vi "move.vi"(8 "error in":errorcluster, 9 "Relative? (T)":bool=TRUE, 10 "Destination (steps)":i16, 11 "Picomotor in":refnum<class "Picomotor.lvclass">) -> (0 "error out":errorcluster, 3 "Picomotor out":refnum<class "Picomotor.lvclass">)   [LabVIEW 2020, in "Picomotor.lvclass"]
uses:
  Picomotor.lvclass
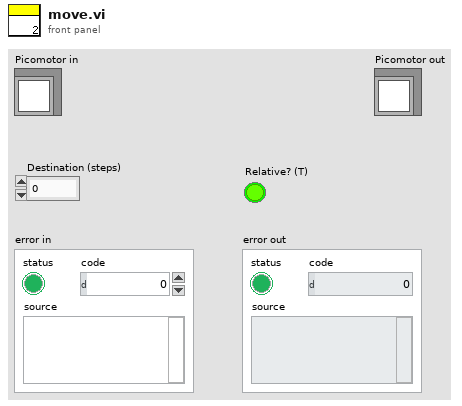
[diagram p1: front panel]
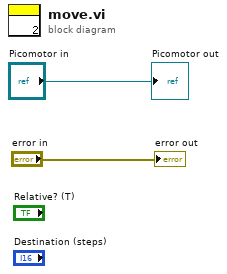
[diagram p0: block diagram]
diagram:
  "Picomotor out" <- "Picomotor in"
  "error out" <- "error in"
